vi "Get Pin Map ID for Sequence.vi"(8 "error in":errorcluster, 11 "sequence context in":refnum<k7>) -> (0 "error out":errorcluster, 2 "pin map id":string, 3 "sequence context out":refnum<k7>)   [LabVIEW 2020, in "MeasurementLink Pin Map.lvlib"]
doc: "Gets the pin map ID for a TestStand sequence."
uses:
  MeasurementLink Pin Map.lvlib
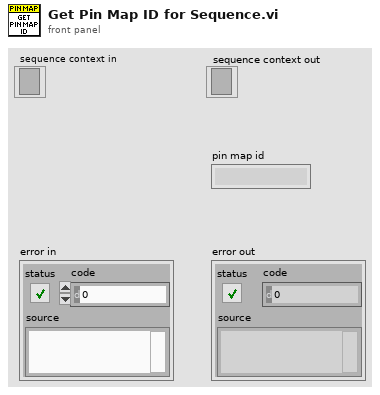
[diagram p1: front panel]
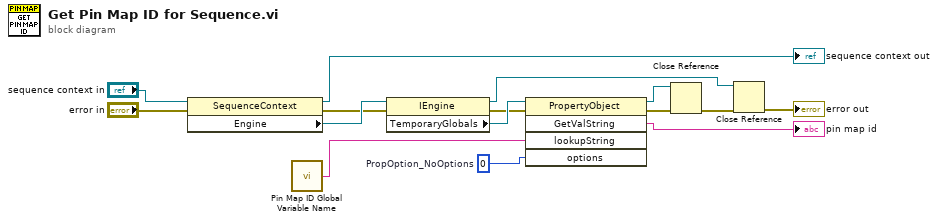
[diagram p0: block diagram]
diagram:
  w7 = 0  # PropOption_NoOptions
  n1 = property class="SequenceContext"(reference="sequence context in", error in="error in") -> (reference out=→"sequence context out":refnum<k7>, error out=w9:errorcluster, "Engine"=w10:refnum<k7>)
  n2 = call "Pin Map ID Global Variable Name.vi"() -> ("global variable name"=w1:string)
  n3 = property class="IEngine"(reference=w10, error in=w9) -> (reference out=w14:refnum<k7>, error out=w8:errorcluster, "TemporaryGlobals"=w11:refnum<k7>)
  n4 = invoke class="PropertyObject" method="GetValString"(reference=w11, error in=w8, "lookupString"=w1, "options"=w7) -> (reference out=w12:refnum<k7>, error out=w13:errorcluster, "GetValString"=→"pin map id":string)  [unwired: 1 in, 2 out]
  n5 = Close Reference(reference=w12, error in (no error)=w13) -> (error out=w15:errorcluster)
  n6 = Close Reference(reference=w14, error in (no error)=w15) -> (error out=→"error out":errorcluster)
